vi "TimeIntToTimeHMSs.vi"(7 "Time Int":u32) -> (4 "Milliseconds":u32, 6 "Seconds":u32, 8 "Minutes":u32, 10 "Hours":u32, 15 "Day":u32)   [LabVIEW 2009]
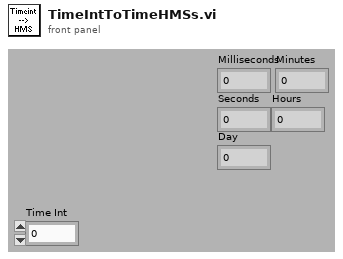
[diagram p1: front panel]
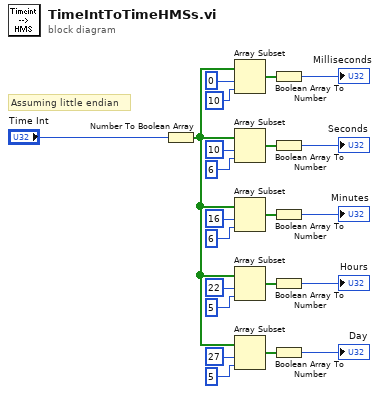
[diagram p0: block diagram]
diagram:
  # "Assuming little endian"
  n1 = Number To Boolean Array(number="Time Int") -> (Boolean array=w6:bool[])
  n2 = Array Subset(array=w6, index=0, length=10) -> (w20:bool[])
  n3 = Array Subset(array=w6, index=10, length=6) -> (w16:bool[])
  n4 = Array Subset(array=w6, index=16, length=6) -> (w14:bool[])
  n5 = Array Subset(array=w6, index=22, length=5) -> (w8:bool[])
  n6 = Array Subset(array=w6, index=27, length=5) -> (w3:bool[])
  n7 = Boolean Array To Number(Boolean array=w20) -> (number=→"Milliseconds":u32)
  n8 = Boolean Array To Number(Boolean array=w16) -> (number=→"Seconds":u32)
  n9 = Boolean Array To Number(Boolean array=w14) -> (number=→"Minutes":u32)
  n10 = Boolean Array To Number(Boolean array=w8) -> (number=→"Hours":u32)
  n11 = Boolean Array To Number(Boolean array=w3) -> (number=→"Day":u32)
